vi "FG Client Library.vi"(1 "FG Action (Read)":T3, 2 "Client Records in":T1[](array[typedef])) -> (0 "Client Records out":T1[](array[typedef]))   [LabVIEW 2011]
uses:
  cRIO/Functional Global Variables/Actions for FG's.ctl
  Source ID Network Location Pair.ctl
  UDP Lib/UDP Network Location.ctl
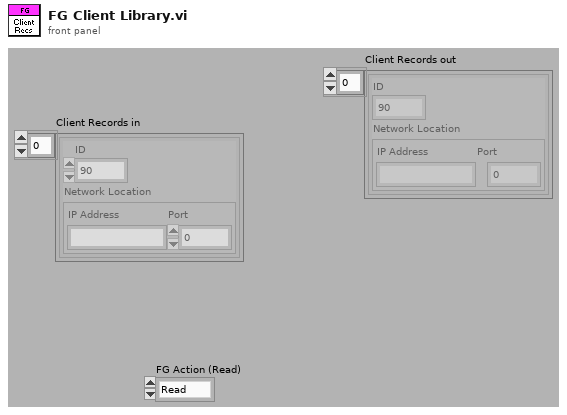
[diagram p1: front panel]
types:
  T1 = typedef "Source ID Network Location Pair.ctl" = cluster{"ID":u32, "Network Location":T2}
  T2 = typedef "UDP Network Location.ctl" = cluster{"IP Address":string, "Port":u16}
  T3 = typedef "Actions for FG's.ctl" = enum16{"Read", "Write"}
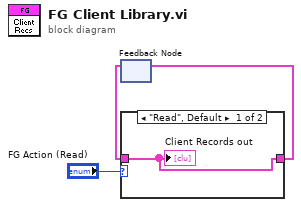
[diagram p0: block diagram]
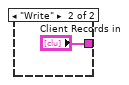
[diagram p2: hidden frame]
diagram:
  n1 = feedback #1() -> (w2:T1[])  [unwired: 1 in]
  n2 = case shown="\"Read\", Default" "FG Action (Read)" {
    tunnel: w2 -> [w4 _]
    tunnel: [w4 "Client Records in"] -> w3
    frame "Read", Default {
      "Client Records out" <- w4
    }
    frame "Write" {
    }
  }
  n3 = feedback-in #1(w3) -> ()
